vi "Convert Thermistor Reading (multiple channels).vi"(0 "Temperature Units (C)":u16(ring) items=["Celsius", "Fahrenheit", "Kelvin", "Rankine"], 6 "Voltage Array":waveform(dbl)[](array[waveform]), 8 "Fit Coefficients":dbl[][](array[numeric]), 10 "Excitation Current":sgl=0.0001 format="%0.2e") -> (2 "Rt Array":dbl[](array[numeric]), 3 "Temperature Array":dbl[](array[numeric]))   [LabVIEW 2019, in "Analysis.lvlib"]
doc: "Converts a thermistor voltage into a temperature. This VI has different modes of operation for voltage-excited and current-excited thermistors. Wire data to the <B>Voltage</B> input to determine the polymorphic instance to use or manually select the instance."
uses:
  Analysis.lvlib
  <vilib>/measure/madcrms.llb/Basic Averaged DC-RMS for N Chan.vi
  <vilib>/measure/NI_MAPro.lvlib
panel:
  in  "Type of Excitation":u16(ring)=1 items=["Voltage Reference", "Current Reference"]
  in  "R1":sgl=5000.0 format="%0.2f"
  in  "Vref":sgl=2.5 format="%0.2f"
  # "Common Applications:  \n{Rt is the thermistor located in the isothermal terminal block. a, b and c are specific for the particular thermistor.}\n\nVoltage Source:\nFor our calculations, R1 is 5kOhms, Rt (Resistance for the thermistor) at 25 degrees Celsius is 5 kOhms, and Vref = 2.5V.\nThe calculated temperature (T) is in Kelvin and is converted to Celsius.\n\nCurrent Source:\nThe DAQPad MIO-16XE-50 card, for example, provides a constant current source at 100 micro Amps, which can be used to excite the thermistor.\n\nIn this case It = 100 micro Amps and Rt at 250 degrees Celsius is 30kOhms with Vo = 0.5V.\n\nNI 435x (Temperature) Devices:\nThe built-in CJC sensor on the 435x accessories is a thermistor.\nHowever, the ConvertThermocouple Reading VI assumes that a thermistor CJC sensor uses voltage excitation.\nThe thermistor on the accessory is read in Ohms mode for greater accuracy, and by playing a trick on the Convert Thermistor Reading VI, we can get an IC Sensor equivalent voltage so that the Convert Thermocouple Reading VI can convert the reading to a temperature."
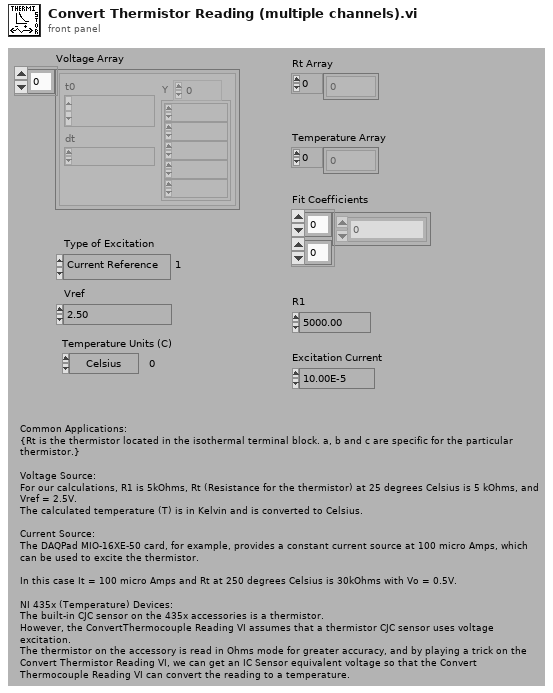
[diagram p1: front panel]
types:
  T1 = enum16{"Rectangular (none)", "Hanning", "Low side lobe"}
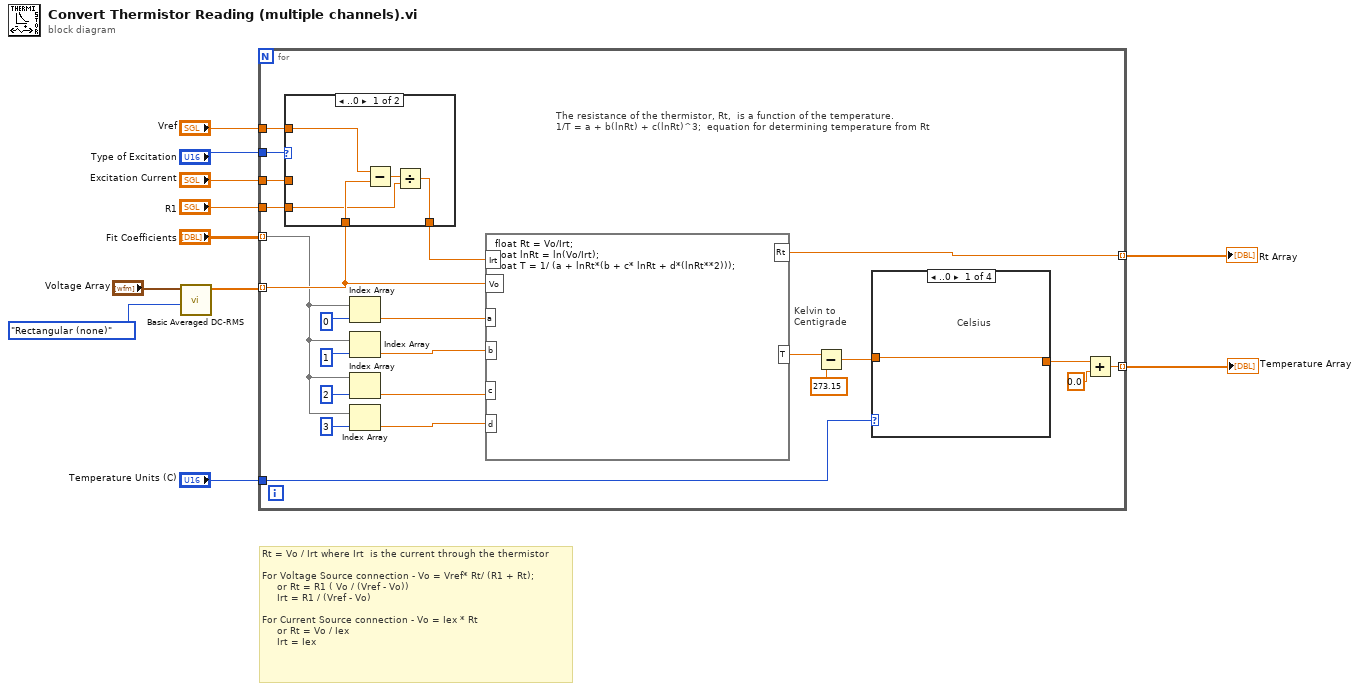
[diagram p0: block diagram]
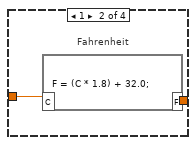
[diagram p2: hidden frame]
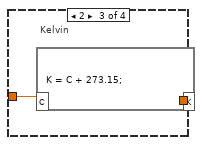
[diagram p3: hidden frame]
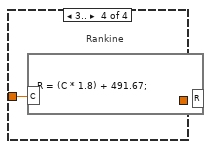
[diagram p4: hidden frame]
diagram:
  # "Rt = Vo / Irt where Irt  is the current through the thermistor\n\nFor Voltage Source connection - Vo = Vref* Rt/ (R1 + Rt); \n     or Rt = R1 ( Vo / (Vref - Vo))\n     Irt = R1 / (Vref - Vo)\n\nFor Current Source connection - Vo = Iex * Rt\n     or Rt = Vo / Iex\n     Irt = Iex"
  n1 = call-poly <vilib>:"Basic Averaged DC-RMS.vi"("window"=T1."Rectangular (none)", "signals in"="Voltage Array") -> ("DC values"=w4:dbl[])  [unwired: 6 in, 3 out]
  n2 = for {
    tunnel: "Type of Excitation" -> [w31]
    tunnel: [w17] -> w2 mode=indexing
    tunnel: w4 -> [w29] mode=indexing
    tunnel: "Fit Coefficients" -> [w12] mode=indexing
    tunnel: [w28] -> w9 mode=indexing
    tunnel: "Excitation Current" -> [w27]
    tunnel: "Vref" -> [w26]
    tunnel: "R1" -> [w25]
    tunnel: "Temperature Units (C)" -> [w24]
    # "The resistance of the thermistor, Rt,  is a function of the temperature.\n1/T = a + b(lnRt) + c(lnRt)^3;  equation for determining temperature from Rt"
    # "Kelvin to \nCentigrade"
    n3 = case shown="..0" w31 {
      tunnel: [w45 w47] -> w32
      tunnel: w29 -> [w44 _]
      tunnel: w27 -> [_ w47]
      tunnel: w26 -> [w43 _]
      tunnel: w25 -> [w42 _]
      frame ..0 {
        n4 = Subtract(x=w43, y=w44) -> (x-y=w46:dbl)
        n5 = Divide(x=w46, y=w42) -> (x/y=w45:dbl)
      }
      frame 1.. {
      }
    }
    n6 = Index Array(array=w12, index=0 ("index (row)")) -> (element=w21:dbl)
    n7 = Index Array(array=w12, index=1 ("index (row)")) -> (element=w20:dbl)
    n8 = Index Array(array=w12, index=2 ("index (row)")) -> (element=w13:dbl)
    n9 = Index Array(array=w12, index=3 ("index (row)")) -> (element=w15:dbl)
    n10 = formula code="float Rt = Vo/Irt;\nfloat lnRt = ln(Vo/Irt);\nfloat T = 1/ (a + lnRt*(b + c* lnRt + d*(lnRt**2)));"("Vo"=w29, "a"=w21, "b"=w20, "c"=w13, "Irt"=w32, "d"=w15) -> ("T"=w34:dbl, "Rt"=w28:dbl)
    n11 = Subtract(x=w34, y=273.15) -> (x-y=w30:dbl)
    n12 = case shown="..0" w24 {
      tunnel: w30 -> [w35 w37 w39 w41]
      tunnel: [w35 w36 w38 w40] -> w18
      frame ..0 {
        # "Celsius"
      }
      frame 1 {
        # "Fahrenheit"
        n13 = formula code="F = (C * 1.8) + 32.0;"("C"=w37) -> ("F"=w36:dbl)
      }
      frame 2 {
        # "Kelvin"
        n14 = formula code="K = C + 273.15;"("C"=w39) -> ("K"=w38:dbl)
      }
      frame 3.. {
        # "Rankine"
        n15 = formula code="R = (C * 1.8) + 491.67;"("C"=w41) -> ("R"=w40:dbl)
      }
    }
    n16 = Add(x=w18, y=0.0) -> (x+y=w17:dbl)
  }
  "Rt Array" <- w9
  "Temperature Array" <- w2
